vi "Simple Server - Front Panel.vi"() -> ()   [LabVIEW 2011]
panel:
  out "Process Variable":string caption="Process Variable Created (Numeric Only)"
  in  "Exit":bool
  out "Value History":dbl(graph)
  out "Value":dbl(knob) scale=0.0..10.0
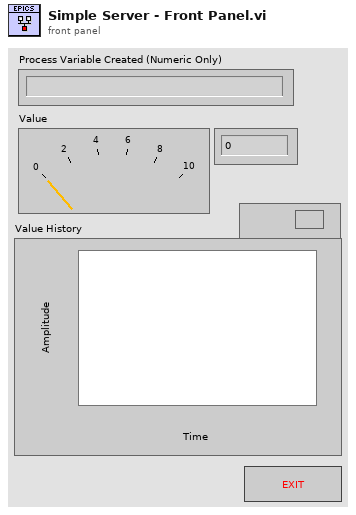
[diagram p1: front panel]
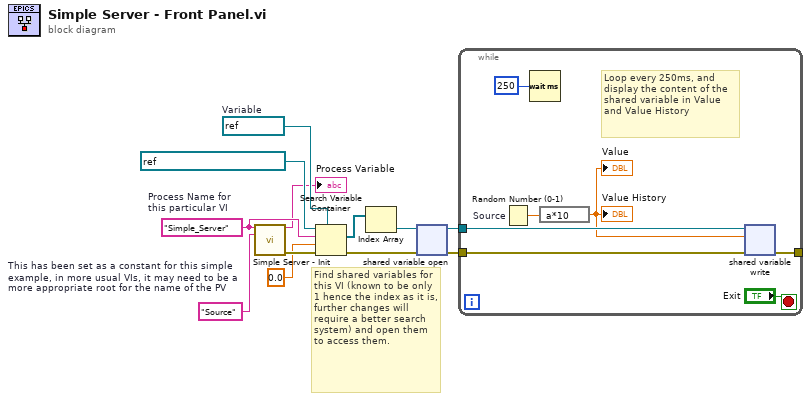
[diagram p0: block diagram]
diagram:
  w1 = "Source"  # This has been set as a constant for this simple example, in more usual VIs, it may need to be a more appropriate root for the name of the PV
  w5 = refnum<k21> refnum  # Variable
  w3 = "Simple_Server"  # Process Name for this particular VI
  # "Find shared variables for this VI (known to be only 1 hence the index as it is, further changes will require a better search system) and open them to access them."
  n1 = call "Simple Server - Init.vi"("Process Name for\nthis particular VI"=w3, "Source"=w1) -> ("Process Variable"=→"Process Variable":string, "error out"=w12:errorcluster)  [unwired: 12 in]
  n2 = Search Variable Container(7:w5, 8:w12, 9:0.0, 10:w3, 11:refnum<k21> "ni.var.psp://localhost/" ("container refnum in")) -> (0:w10:errorcluster, 2:w7:refnum<k21>[])  [unwired: 1 in, 1 out]
  n3 = Index Array(array=w7) -> (element=w9:refnum<k21>)  [unwired: 1 in]
  n4 = shared-variable-open(w9, w10) -> (w8:refnum<k21>, w11:errorcluster)  [unwired: 1 in]
  n5 = while {
    tunnel: w8 -> [w17]
    tunnel: w11 -> [w16]
    tunnel: [w15] -> _
    stop <- "Exit" stop-if-true
    # "Loop every 250ms, and display the content of the shared variable in Value and Value History"
    n6 = Random Number (0-1) "Source"() -> (number: 0 to 1=w14:dbl)
    n7 = Wait (ms)(milliseconds to wait=u32 250) -> ()  [unwired: 1 out]
    n8 = expression code="a*10"(w14) -> (w13:dbl)
    "Value" <- w13
    "Value History" <- w13
    n9 = shared-variable-write(w17, w16, w13) -> (w15:errorcluster)  [unwired: 1 out]
  }
